vi "hasPacketIdentifier.vi"(11 "SUBACK in":refnum<class "SUBACK.lvclass">) -> (2 "Has Packet Identifier":bool, 3 "SUBACK out":refnum<class "SUBACK.lvclass">)   [LabVIEW 2013, in "MQTT_Control_Packets.lvlib" / "SUBACK.lvclass"]
uses:
  SUBACK.lvclass
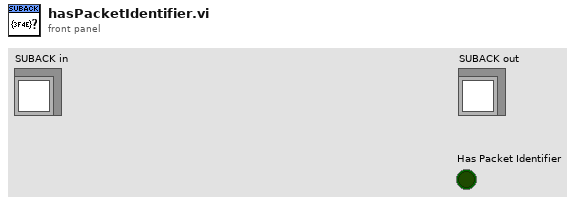
[diagram p1: front panel]
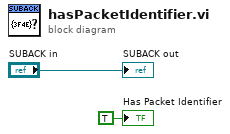
[diagram p0: block diagram]
diagram:
  "SUBACK out" <- "SUBACK in"
  "Has Packet Identifier" <- TRUE ("As Packet Identifier")
